vi "DealResultVi.vi"(4 "Multicolumn Listbox":i32(listbox), 5 "Event Data":cluster{"uiMsg":refnum<k7>, "cancel":bool}, 6 "Control Ref":refnum<k7>, 7 "Event Common Data":T1) -> (1 "Event Data Out":cluster{"cancel":bool})   [LabVIEW 2018]
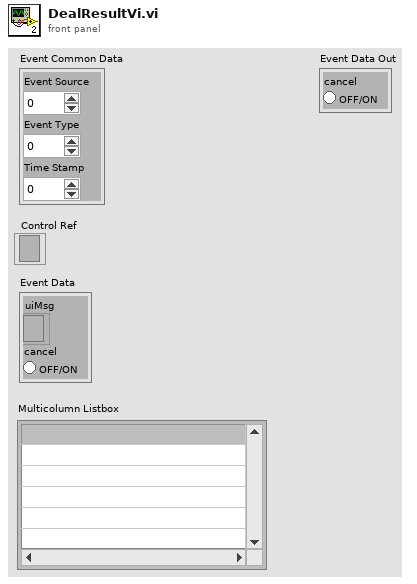
[diagram p1: front panel]
types:
  T1 = cluster{"Event Source":i32, "Event Type":u32, "Time Stamp":u32}
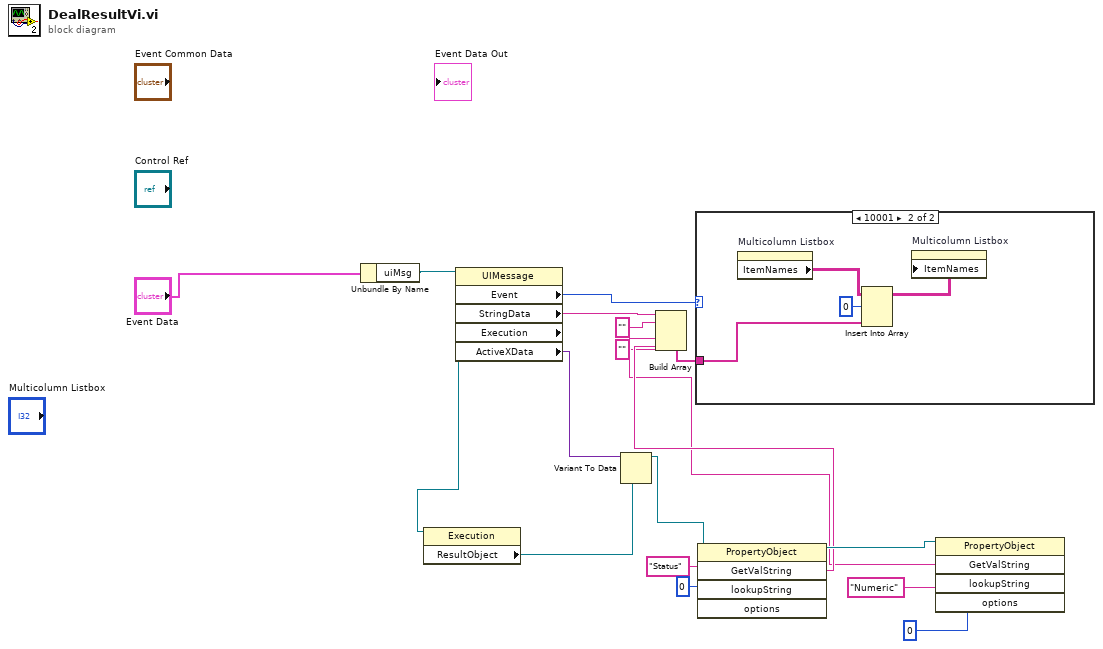
[diagram p0: block diagram]
diagram:
  n1 = Unbundle By Name("Event Data") -> ("uiMsg"=w18:refnum<k7>)
  n2 = property class="UIMessage"(reference=w18) -> ("Event"=w17:i32, "StringData"=w6:string, "Execution"=w11:refnum<k7>, "ActiveXData"=w14:variant)  [unwired: 1 in, 2 out]
  n3 = property class="Execution"(reference=w11) -> ("ResultObject"=w10:refnum<k7>)  [unwired: 1 in, 2 out]
  n4 = Variant To Data(type=w10, Variant=w14) -> (data=w16:refnum<k7>)  [unwired: 1 in, 1 out]
  n5 = invoke class="PropertyObject" method="GetValString"(reference=w16, "lookupString"="Status", "options"=0) -> (reference out=w7:refnum<k7>, "GetValString"=w5:string)  [unwired: 2 in, 3 out]
  n6 = invoke class="PropertyObject" method="GetValString"(reference=w7, "lookupString"="Numeric", "options"=0) -> ("GetValString"=w4:string)  [unwired: 2 in, 4 out]
  n7 = Build Array(w6, "" ("element"), "" ("element"), w4, w5) -> (w3:string[])
  n8 = case shown="10001" w17 {
    tunnel: w3 -> [_ w20]
    frame 0, Default {
    }
    frame 10001 {
      n9 = property on="Multicolumn Listbox" class="MCListbox (strict)"() -> ("ItemNames"=w22:string[][])  [unwired: 2 in, 2 out]
      n10 = Insert Into Array(array=w22, index (row)=0, new element=w20) -> (w21:string[][])  [unwired: 1 in]
      n11 = property on="Multicolumn Listbox" class="MCListbox (strict)"("ItemNames"=w21) -> ()  [unwired: 2 in, 2 out]
    }
  }
